vi "Target Stuff V.5.0.vi"(8 "Left Joystick Y":dbl, 9 "Right Joystick Y":dbl, 10 "Target Y":dbl, 11 "Target X":dbl) -> (2 "Left Motor":dbl, 3 "Right Motor":dbl)   [LabVIEW 2016]
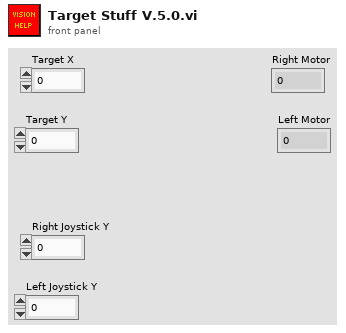
[diagram p1: front panel]
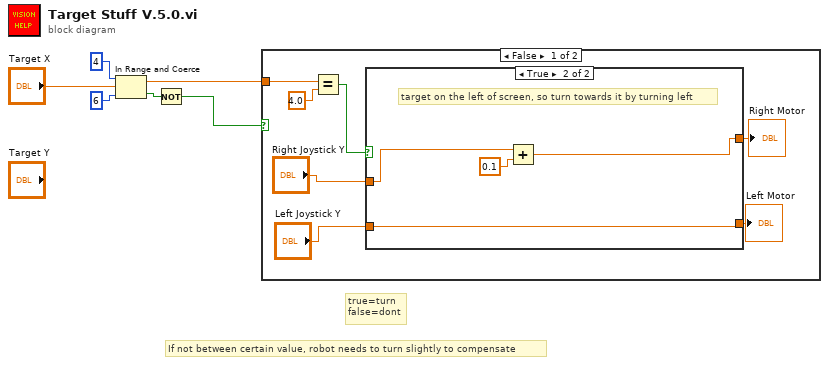
[diagram p0: block diagram]
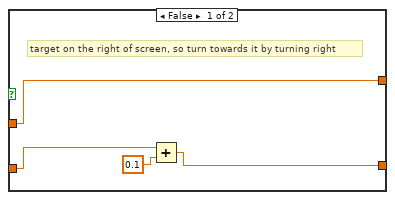
[diagram p2: hidden frame]
diagram:
  # "true=turn\nfalse=dont"
  # "If not between certain value, robot needs to turn slightly to compensate"
  n1 = In Range and Coerce(upper limit=4, x="Target X", lower limit=6) -> (coerced(x)=w1:dbl, In Range?=w3:bool)
  n2 = Not(x=w3) -> (.not. x?=w2:bool)
  n3 = case shown="False" w2 {
    tunnel: w1 -> [w13 _]
    frame False {
      n4 = Equal?(x=w13, y=4.0) -> (x = y?=w9:bool)
      n5 = case shown="True" w9 {
        tunnel: [w14 w19] -> w11
        tunnel: [w15 w18] -> w10
        tunnel: "Right Joystick Y" -> [w14 w20]
        tunnel: "Left Joystick Y" -> [w16 w18]
        frame False {
          # "target on the right of screen, so turn towards it by turning right"
          n6 = Add(x=w16, y=0.1) -> (x+y=w15:dbl)
        }
        frame True {
          # "target on the left of screen, so turn towards it by turning left"
          n7 = Add(x=w20, y=0.1) -> (x+y=w19:dbl)
        }
      }
      "Right Motor" <- w11
      "Left Motor" <- w10
    }
    frame True {
    }
  }
